vi "Method_Const.vi"(4 "Value":i8, 5 "Value A":refnum<class "Abs_I8 Integer.lvclass">) -> (1 "Result":refnum<class "Abs_Boolean.lvclass">)   [LabVIEW 2021, in "Greater Equal_I8.lvclass"]
uses:
  Greater Equal_I8.lvclass
  Abs_Types/I8 Integer/Abs_I8 Integer.lvclass
  C:/Program Files (x86)/National Instruments/LabVIEW 2021/vi.lib/TSA/Abstract Data Classes/Abs_Types/Numeric/Abs_Numeric.lvclass
  Abs_Types/Boolean/Abs_Boolean.lvclass
  C:/TSA/LV_Abstract/Source/Functions/Support/Compare/Two Term/I8/AbsComp_Two Term_I8.lvclass
  C:/Program Files (x86)/National Instruments/LabVIEW 2021/vi.lib/TSA/Abstract Data Classes/Abs_Types/Boolean/Abs_Boolean.lvclass
  Support/Compare/Two Term/I8/AbsComp_Two Term_I8.lvclass/AbsComp_Two Term_I8.ctl
  Support/Compare/Two Term/I8/Properties/Write Numeric A.vi
  Support/Compare/Two Term/I8/Properties/Write Numeric B.vi
  Constants/Support/I8/Const_I8.lvclass
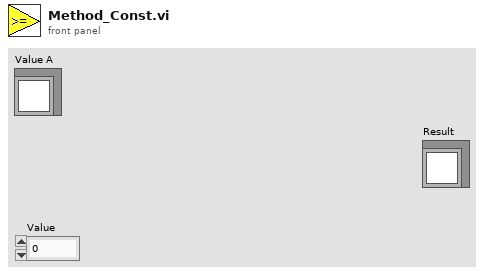
[diagram p1: front panel]
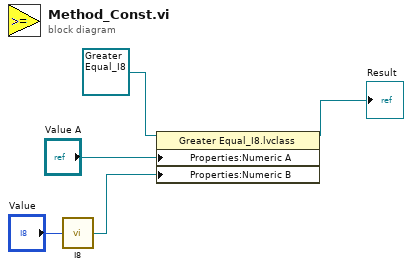
[diagram p0: block diagram]
diagram:
  n1 = call "I8.vi"("Value"="Value") -> ("Constant"=w2:refnum<class "Abs_I8 Integer.lvclass">)  [unwired: 4 in]
  n2 = property class="Greater Equal_I8.lvclass"(reference=refnum<class "Greater Equal_I8.lvclass"> refnum ("Greater 0_U64.lvclass"), "Properties:Numeric A"="Value A", "Properties:Numeric B"=w2) -> (reference out=→"Result":refnum<class "Greater Equal_I8.lvclass">)  [unwired: 1 in, 1 out]
